vi "LabVIEW Project to Additional Installer SBOM Components.vi"(8 "error in (no error)":errorcluster, 10 "Build Specification Name (\"\" = first installer)":string, 11 "LabVIEW Project Path":path) -> (0 "error out":errorcluster, 3 "Installer components":refnum<class "CycloneDX Component.lvclass">[](array[class]))   [LabVIEW 2017, in "LabVIEW Installer Support.lvlib"]
doc: "Reads the 'additional installers' from a LabVIEW project installer build specification and converts it to an array of CycloneDX SBOM components."
uses:
  LabVIEW Installer Support.lvlib
  CycloneDX/CycloneDX Component/CycloneDX Component.lvclass
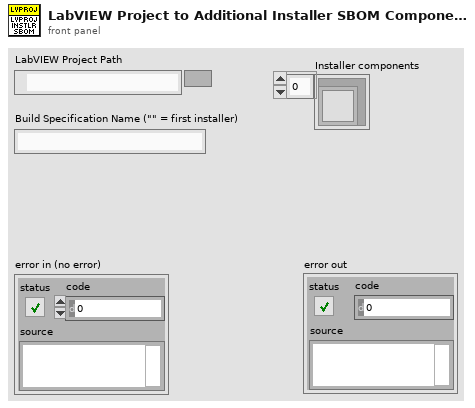
[diagram p1: front panel]
types:
  T1 = typedef "LabVIEW Installer Support.lvlib/Additional Installer.ctl" = cluster{"flavorID":string, "productID":string, "productName":string, "upgradeCode":string, "SoftDeps":T2[]}
  T2 = typedef "LabVIEW Installer Support.lvlib/Installer Soft Dep.ctl" = cluster{"productName":string, "upgradeCode":string, "exclude?":bool}
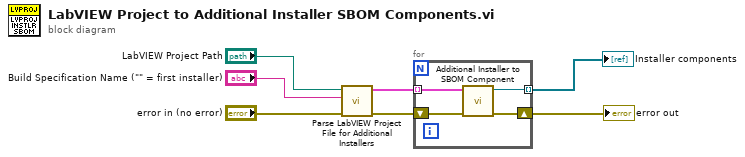
[diagram p0: block diagram]
diagram:
  n1 = call "Parse LabVIEW Project File for Additional Installers.vi"("error in (no error)"="error in (no error)", "Build Specification Name (\"\" = first installer)"="Build Specification Name (\"\" = first installer)", "LabVIEW Project Path"="LabVIEW Project Path") -> ("error out"=w7:errorcluster, "Additional Installers"=w6:T1[])  [unwired: 7 in]
  n2 = for {
    tunnel: w6 -> [w10] mode=indexing
    tunnel: [w9] -> w5 mode=indexing
    shift-right: [w8] -> w4
    shift-left: w7 -> [w11]
    n3 = call "Additional Installer to SBOM Component.vi"("error in (no error)"=w11, "Additional Installer"=w10) -> ("error out"=w8:errorcluster, "LabVIEW installer component out"=w9:refnum<class "CycloneDX Component.lvclass">)  [unwired: 8 in]
  }
  "Installer components" <- w5
  "error out" <- w4
